vi "High Resolution Polling Wait.vi"(8 "error in (no error)":errorcluster, 11 "seconds to wait":dbl format="%#_6p") -> (0 "error out":errorcluster)   [LabVIEW 2021, in "Timer-API.lvlib" / "Timer Session.lvclass"]
uses:
  Timer Session.lvclass
  Timer Session.lvclass/Timer Session.ctl
  kernel32.dll
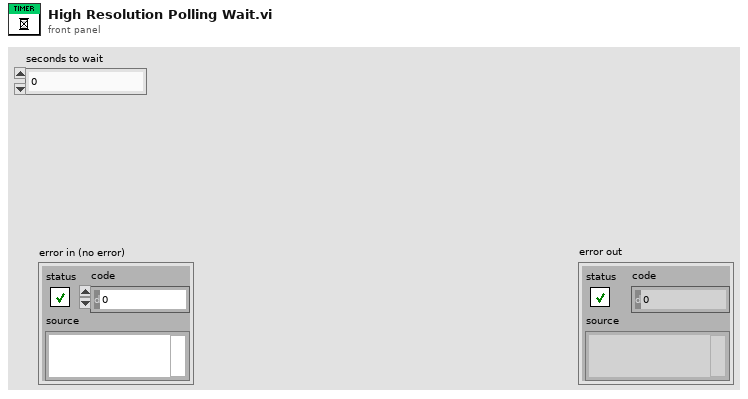
[diagram p1: front panel]
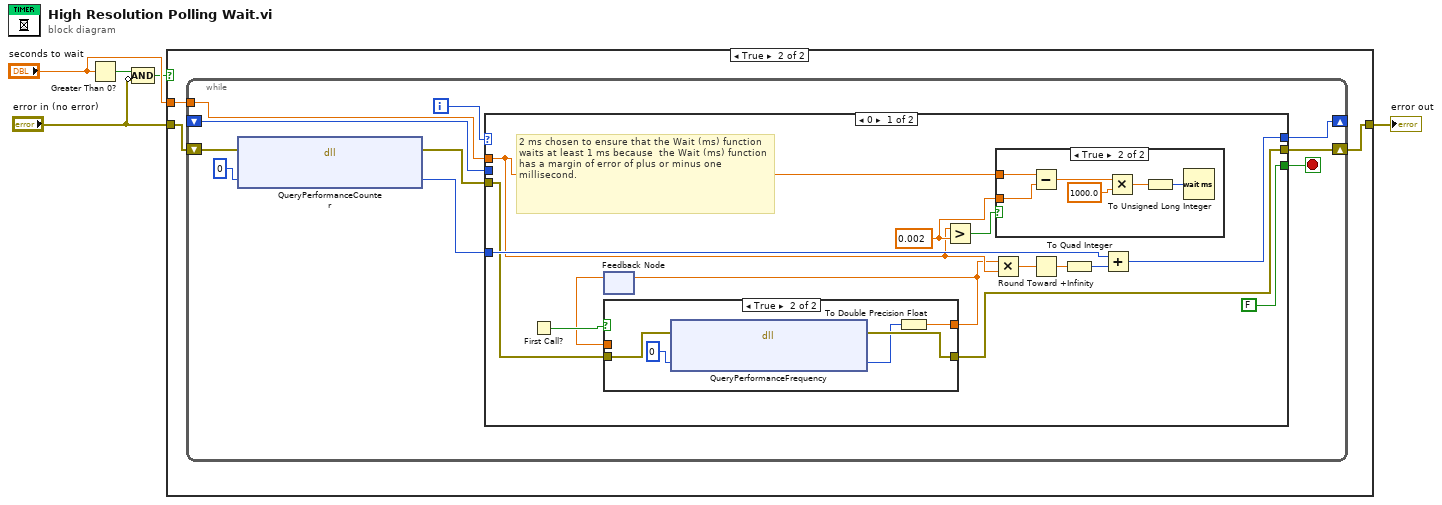
[diagram p0: block diagram]
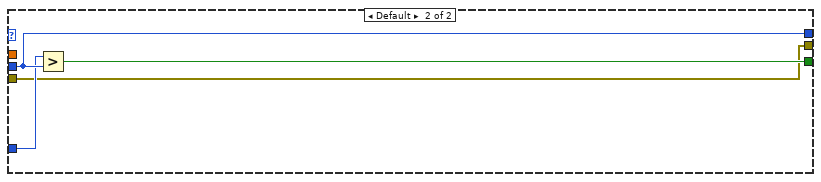
[diagram p5: hidden frame]
diagram:
  n1 = Greater Than 0?(x="seconds to wait") -> (x > 0?=w2:bool)
  n2 = Compound Arithmetic op=AND(w2, invert "error in (no error)") -> (w1:bool)
  n3 = case shown="True" w1 {
    tunnel: "seconds to wait" -> [_ w9]
    tunnel: [w6 w7] -> w5
    tunnel: "error in (no error)" -> [w6 w8]
    frame False {
    }
    frame True {
      n4 = while {
        shift-right: [w18] -> _
        shift-left: _ -> [w19]
        tunnel: w9 -> [w15]
        shift-right: [w11] -> w7
        shift-left: w8 -> [w13]
        i -> [w16]
        stop <- w17 stop-if-true
        n5 = dll-call lib="kernel32.dll" fn="QueryPerformanceCounter"(error in=w13, "lpPerformanceCount"=i64 0) -> (error out=w12:errorcluster, "lpPerformanceCount"=w14:i64)  [unwired: 3 in, 1 out]
        n6 = case shown="0" w16 {
          tunnel: w19 -> [_ w49]
          tunnel: [w33 w49] -> w18
          tunnel: [FALSE w50] -> w17
          tunnel: w15 -> [w25 _]
          tunnel: w14 -> [w29 w48]
          tunnel: w12 -> [w21 w47]
          tunnel: [w20 w47] -> w11
          frame 0 {
            w30 = 0.002 ("y")
            # "2 ms chosen to ensure that the Wait (ms) function waits at least 1 ms because  the Wait (ms) function has a margin of error of plus or minus one millisecond."
            n7 = First Call?() -> (First Call?: T/F=w24:bool)
            n8 = feedback #1() -> (w22:dbl)  [unwired: 1 in]
            n9 = case shown="True" w24 {
              tunnel: w22 -> [w35 _]
              tunnel: [w35 w40] -> w23
              tunnel: w21 -> [w34 w39]
              tunnel: [w34 w38] -> w20
              frame False {
              }
              frame True {
                n10 = dll-call lib="kernel32.dll" fn="QueryPerformanceFrequency"(error in=w39, "lpFrequency"=i64 0) -> (error out=w38:errorcluster, "lpFrequency"=w37:i64)  [unwired: 3 in, 1 out]
                n11 = To Double Precision Float(number=w37) -> (double precision float=w40:dbl)
              }
            }
            n12 = feedback-in #1(w23) -> ()
            n13 = Greater?(x=w25, y=w30) -> (0:w31:bool)
            n14 = Multiply(x=w23, y=w25) -> (x*y=w28:dbl)
            n15 = case shown="True" w31 {
              tunnel: w25 -> [_ w42]
              tunnel: w30 -> [_ w41]
              frame False {
              }
              frame True {
                n16 = Subtract(x=w42, y=w41) -> (x-y=w46:dbl)
                n17 = Multiply(x=w46, y=1000.0) -> (x*y=w43:dbl)
                n18 = To Unsigned Long Integer(number=w43) -> (unsigned 32bit integer=w44:u32)
                n19 = Wait (ms)(milliseconds to wait=w44) -> ()  [unwired: 1 out]
              }
            }
            n20 = Round Toward +Infinity(x=w28) -> (ceil(x): smallest int >= x=w27:dbl)
            n21 = To Quad Integer(1:w27) -> (0:w26:i64)
            n22 = Add(x=w29, y=w26) -> (x+y=w33:i64)
          }
          frame Default {
            n23 = Greater?(x=w48, y=w49) -> (0:w50:bool)
          }
        }
      }
    }
  }
  "error out" <- w5
